vi "02_array_2.vi"(8 "errorIn":errorcluster, 11 "ArrayIn":i32[](array[numeric])) -> (0 "errorOut":errorcluster, 3 "ArrayOut":i32[](array[numeric]))   [LabVIEW 2011]
panel:
  in  "BooleanIn":bool
  out "BooleanOut":bool
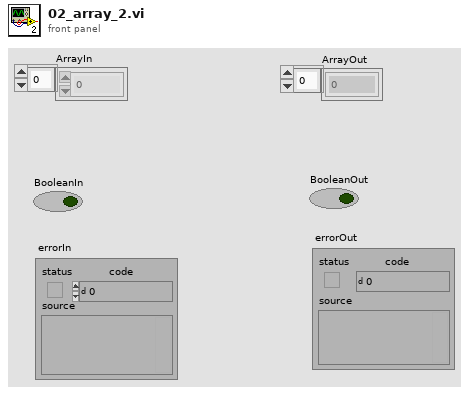
[diagram p1: front panel]
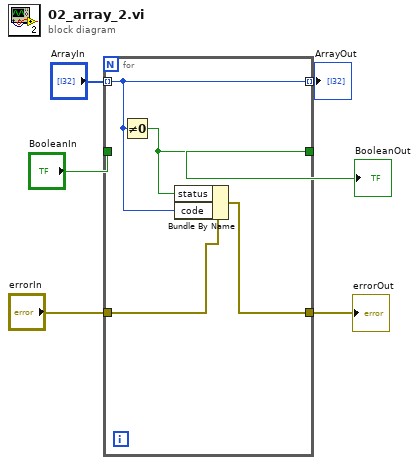
[diagram p0: block diagram]
diagram:
  n1 = for {
    tunnel: "ArrayIn" -> [w7] mode=indexing
    tunnel: [w7] -> w3 mode=indexing
    tunnel: "BooleanIn" -> [_]
    tunnel: [w8] -> w6
    tunnel: "errorIn" -> [w10]
    tunnel: [w9] -> w1
    n2 = Not Equal To 0?(x=w7) -> (x != 0?=w8:bool)
    n3 = Bundle By Name(cluster=w10, "status"=w8, "code"=w7) -> (w9:errorcluster)
  }
  "BooleanOut" <- w6
  "ArrayOut" <- w3
  "errorOut" <- w1
